vi "ColorToObject.vi"(5 "Color":u32(colorbox), 11 "error in (no error)":errorcluster) -> (6 ".Net Color":refnum<k24>, 15 "error out":errorcluster)   [LabVIEW 2018, in "DataGridView.lvclass"]
doc: "Converts a labview color to the .net <b>System.Drawing.Color Object</b>"
uses:
  DataGridView.lvclass
  System.Drawing
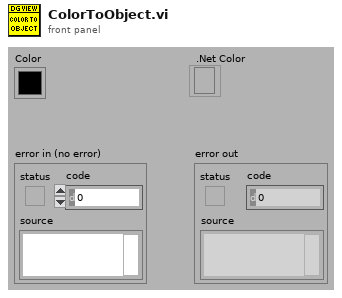
[diagram p1: front panel]
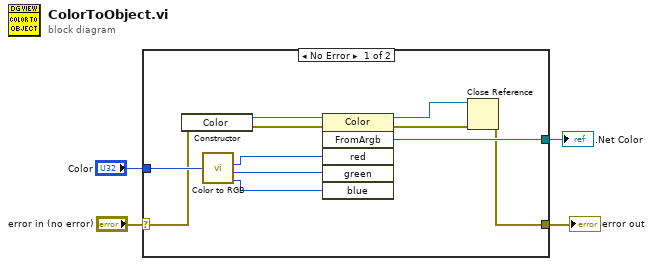
[diagram p0: block diagram]
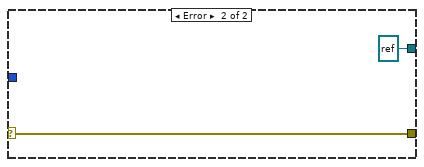
[diagram p2: hidden frame]
diagram:
  n1 = case shown="No Error" "error in (no error)" {
    selector: "error in (no error)" -> [w6 w17]
    tunnel: [w5 w17] -> w3
    tunnel: "Color" -> [w10 _]
    tunnel: [w9 refnum<k24> refnum ("FromArgb")] -> w1
    frame No Error {
      n2 = constructor class="Color"(error in=w6) -> (reference out=w15:refnum<k24>, error out=w11:errorcluster)  [unwired: 2 in, 1 out]
      n3 = call <vilib>:"Color to RGB.vi"("Color"=w10) -> ("R"=w14:u8, "G"=w13:u8, "B"=w12:u8)  [unwired: 1 out]
      n4 = invoke class="Color" method="FromArgb"(reference=w15, error in=w11, "red"=w14, "green"=w13, "blue"=w12) -> (reference out=w8:refnum<k24>, error out=w7:errorcluster, "FromArgb"=w9:refnum<k24>)  [unwired: 1 in, 3 out]
      n5 = Close Reference(reference=w8, error in (no error)=w7) -> (error out=w5:errorcluster)
    }
    frame Error {
    }
  }
  "error out" <- w3
  ".Net Color" <- w1
